vi "SV TDMS Read Spectrum Info.vi"(0 "tdms file":refnum<k34>, 5 "group name in":string, 7 "channel name in":string, 11 "error in":errorcluster) -> (4 "tdms file out":refnum<k34>, 6 "group name out":string, 8 "channel name out":string, 14 "spectrum info":T1 {"x-axis units" items=["Time (s)"=0, "Frequency-CB (Hz)"=1, "Frequency-CPB (Hz)"=1248, "Frequency-Arbitrary (Hz)"=2357, "Quefrency (s)"=2, "Revolutions (rev)"=3, "Order"=4, "Speed (RPM)"=11, "Speed (rad/s)"=21, "Index"=65535]; "weighting filter" items=["Linear", "A-weighting", "B-weighting", "C-weighting", "ITU-R 468-4", "Dolby", "CCITT", "C-message", "Wb", "Wc", "Wd", "We", "Wf", "Wh", "Wj", "Wk", "Wm", "AES17 20 kHz lowpass", "AES17 40 kHz lowpass", "AES17 20 kHz highpass", "AES17 40 kHz highpass"]; "dB reference [EU]" format="%.2f"; "engineering units" items=["custom..."=0, "V"=1, "A"=21, "C"=30, "pC"=31, "s"=32, "-"=29, "Pa"=2, "N"=20, "g"=3, "m/s^2"=4, "m/s"=5, "m"=6, "mm/s"=12, "mm"=13, "micron/s"=14, "micron"=15, "in/s^2"=7, "in/s"=8, "in"=9, "mil/s"=10, "mil"=11, "rad/s^2"=16, "rad/s"=17, "rad"=18, "deg/s^2"=26, "deg/s"=27, "deg"=28, "RPM"=22, "cycle/s^2"=23, "Hz"=24, "cycle"=25, "strain"=19]; "spectral info"."window" items=["None "=0, "Hanning"=1, "Hamming"=2, "Blackman-Harris"=3, "Exact Blackman"=4, "Blackman"=5, "Flat Top"=6, "4 Term B-Harris "=7, "7 Term B-Harris"=8, "Low Sidelobe"=9, "Force - Exponential"=10, "Gaussian"=62]}, 15 "error out":errorcluster)   [LabVIEW 2017]
uses:
  <vilib>/addons/_NISVFA/_Shared subVIs/Controls/svc_Spectrum Info.ctl
  <vilib>/addons/_NISVFA/_Shared subVIs/Controls/svc_X-Axis Units.ctl
  <vilib>/addons/_NISVFA/_Shared subVIs/Controls/svc_Spectrum Type.ctl
  <vilib>/addons/_NISVFA/_Shared subVIs/Controls/svc_Engineering Units Text Ring.ctl
  <vilib>/addons/_NISVFA/_Shared subVIs/Controls/svc_Weighting Filter Text Ring.ctl
  <vilib>/addons/_NISVFA/_Shared subVIs/Controls/svc_Complimentary Spectrum Units.ctl
  <vilib>/addons/_NISVFA/_Shared subVIs/Controls/NI Channel Properties.ctl
  <vilib>/addons/_NISVFA/_Shared subVIs/Controls/SV Channel Properties.ctl
  <vilib>/addons/_NISVFA/_Shared subVIs/Common/svc_Get Weighting Enum and Labels.vi
  <vilib>/addons/_NISVFA/_Shared subVIs/Common/svc_Unit Label Lexical Class.vi
  <vilib>/addons/_NISVFA/_Shared subVIs/Common/svc_Format Value (DBL).vi
  <vilib>/addons/_NISVFA/_Shared subVIs/Spectrum Info/sfva_Get SV Info from Spectrum Info Description.vi
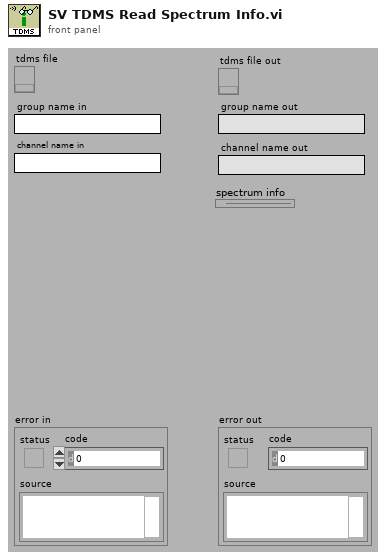
[diagram p1: front panel]
types:
  T1 = typedef "svc_Spectrum Info.ctl" = cluster{"channel name":string, "description":string, "x-axis units":T2, "spectral info":cluster{"spectrum type":T3, "linear/dB":enum16{"linear", "dB"}, "window":u16, "window size":i32, "FFT size":i32}, "engineering units":T4, "custom label":string, "dB reference [EU]":dbl, "peak units":enum16{"rms", "peak", "peak-peak"}, "weighting filter":T5, "spectral density?":bool, "unit label":string, "spectrum skewed?":bool, "complimentary spectrum units":T6}
  T2 = typedef "svc_X-Axis Units.ctl" = u16
  T3 = typedef "svc_Spectrum Type.ctl" = enum16{"FFT Spectrum [complex]", "Amplitude [Magnitude]", "Power [Magnitude^2]", "Cross Spectrum [complex]", "Frequency Response [Complex]"}
  T4 = typedef "svc_Engineering Units Text Ring.ctl" = u16
  T5 = typedef "svc_Weighting Filter Text Ring.ctl" = u16
  T6 = typedef "svc_Complimentary Spectrum Units.ctl" = enum16{"none", "radians", "degrees", "cycles", "imaginary"}
  T7 = typedef "NI Channel Properties.ctl" = u16
  T8 = typedef "NI Function Info.ctl" = cluster{"function type":T9, "function subtype":T10, "X-dimension":T2}
  T9 = typedef "NI Function Type.ctl" = u16
  T10 = typedef "NI Function SubType.ctl" = u16
  T11 = enum16{"No averaging", "Vector averaging", "RMS averaging", "Peak hold"}
  T12 = typedef "SV Channel Properties.ctl" = u16
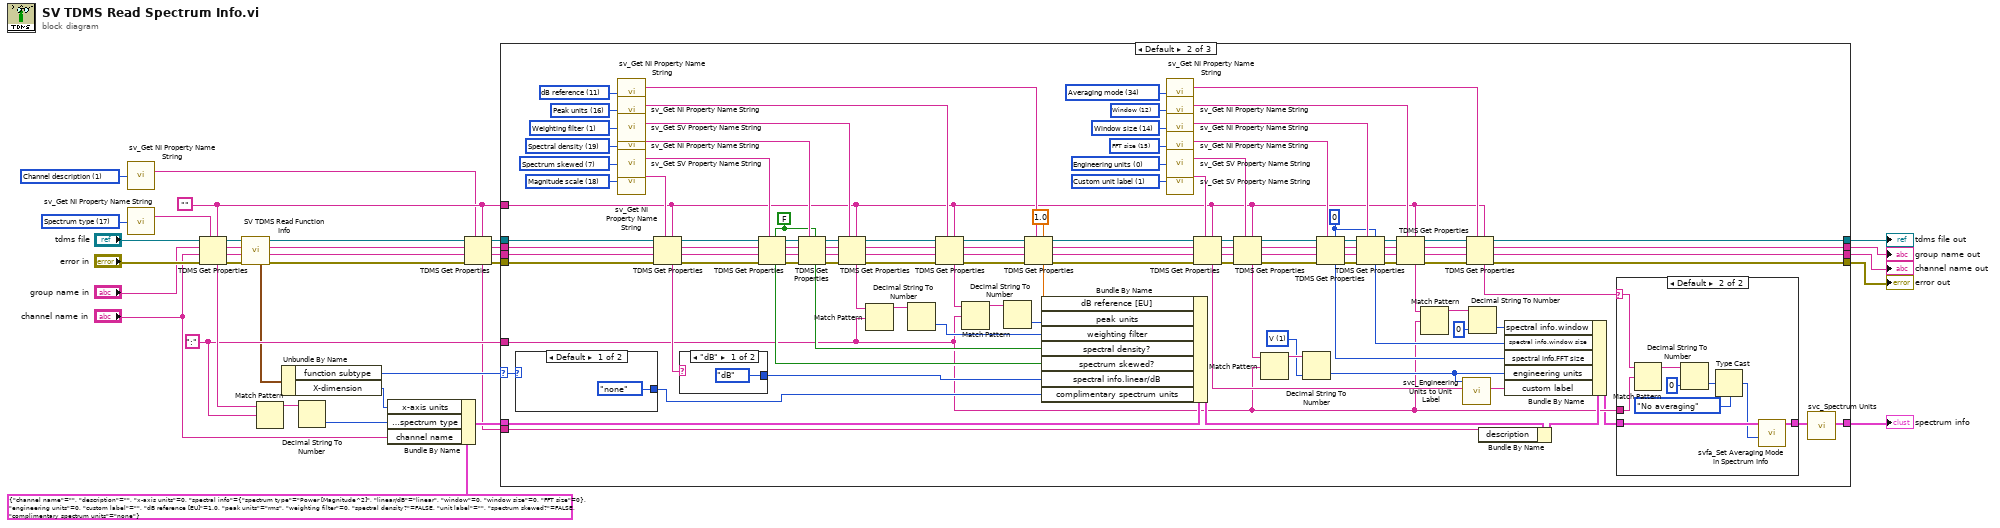
[diagram p0: block diagram]
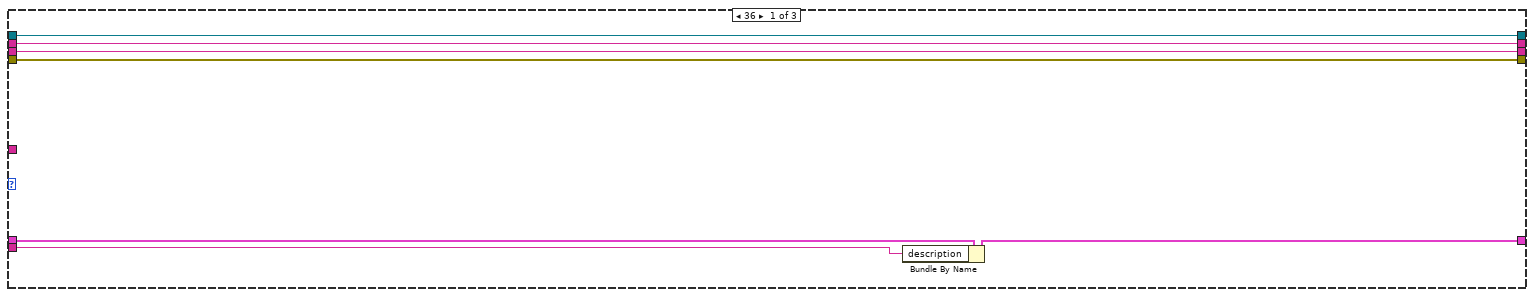
[diagram p2: hidden frame]
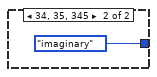
[diagram p4: hidden frame]
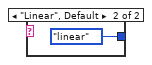
[diagram p5: hidden frame]
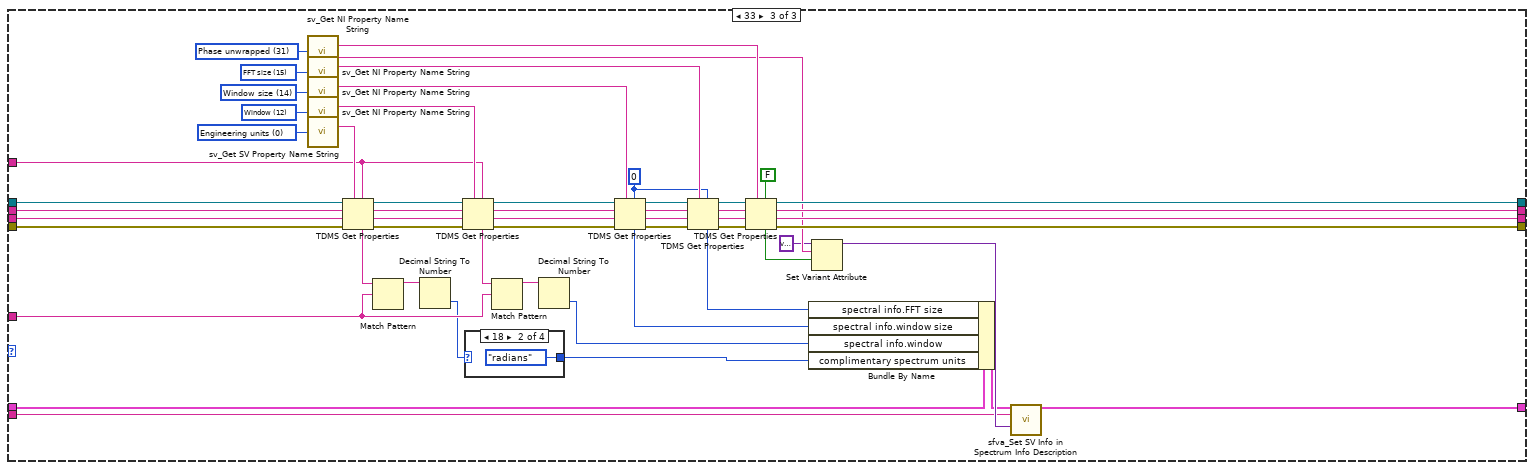
[diagram p6: hidden frame]
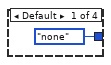
[diagram p7: hidden frame]
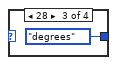
[diagram p8: hidden frame]
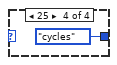
[diagram p9: hidden frame]
diagram:
  w6 = T7 1 items=["Channel name", "Channel description", "Axis label", "Unit string", "Waveform X-axis label", "Waveform X-axis unit string", "x0", "dx", "Number of samples", "X channel", "Filter settled", "dB reference", "Window", "Window parameter", "Window size", "FFT size", "Peak units", "Spectrum type", "Magnitude scale", "Spectral density", "Sensor sensitivity (mV/EU)", "X-axis dimension", "LabVIEW datatype", "Function type", "Function subtype", "X values", "Independent channel", "Column index", "Collection name", "Collection ID", "X Columns", "Phase unwrapped"] ("property")
  w18 = ":" ("regular expression")
  w7 = "" ("TDMS property name")
  w32 = T7 17 items=["Channel name", "Channel description", "Y-axis label", "Y-axis unit string", "X-axis label", "X-axis unit string", "x0", "dx", "Number of samples", "X channel", "Filter settled", "dB reference", "Window", "Window parameter", "Window size", "FFT size", "Peak units", "Spectrum type", "Magnitude scale", "Spectral density"] ("property")
  n1 = call <vilib>:"sv_Get NI Property Name String.vi"("property"=w6) -> ("TDMS property name"=w5:string)  [unwired: 13 in, 1 out]
  n2 = call <vilib>:"sv_Get NI Property Name String.vi"("property"=w32) -> ("TDMS property name"=w31:string)  [unwired: 13 in, 1 out]
  n3 = TDMS Get Properties(5:w7, 7:w31, 8:"error in", 9:"channel name in", 10:"group name in", 11:"tdms file") -> (0:w21:errorcluster, 1:w20:string, 2:w19:string, 3:w22:refnum<k34>, 4:w30:string)  [unwired: 1 out]
  n4 = call <vilib>:"SV TDMS Read Function Info.vi"("error in (no error)"=w21, "channel name"=w20, "group name"=w19, "tdms file in"=w22) -> ("error out"=w14:errorcluster, "channel name out"=w13:string, "group name out"=w12:string, "tdms file out"=w11:refnum<k34>, "function info"=w17:T8)  [unwired: 2 in, 1 out]
  n5 = Match Pattern(string=w30, regular expression=w18) -> (before substring=w29:string)  [unwired: 1 in, 3 out]
  n6 = Unbundle By Name(w17) -> ("function subtype"=w16:T10, "X-dimension"=w15:T2)
  n7 = Decimal String To Number(string=w29) -> (number=w28:i32)  [unwired: 2 in, 1 out]
  n8 = Bundle By Name(cluster=T1 {"channel name"="", "description"="", "x-axis units"=0, "spectral info"={"spectrum type"=enum."Power [Magnitude^2]", "linear/dB"=enum."linear", "window"=0, "window size"=0, "FFT size"=0}, "engineering units"=0, "custom label"="", "dB reference [EU]"=1.0, "peak units"=enum."rms", "weighting filter"=0, "spectral density?"=FALSE, "unit label"="", "spectrum skewed?"=FALSE, "complimentary spectrum units"=enum."none"} ("spectrum info in"), "x-axis units"=w15, "spectral info.spectrum type"=w28, "channel name"="channel name in") -> (w27:T1)
  n9 = TDMS Get Properties(5:w7, 7:w5, 8:w14, 9:w13, 10:w12, 11:w11) -> (0:w1:errorcluster, 1:w8:string, 2:w9:string, 3:w10:refnum<k34>, 4:w2:string)  [unwired: 1 out]
  n10 = case shown="Default" w16 {
    selector: w16 -> [_ w62 _]
    tunnel: [w43 w52 w185] -> w36
    tunnel: [w42 w53 w184] -> w35
    tunnel: [w41 w54 w183] -> w34
    tunnel: [w40 w55 w182] -> w33
    tunnel: w10 -> [w43 w126 w226]
    tunnel: w9 -> [w42 w127 w225]
    tunnel: w8 -> [w41 w128 w224]
    tunnel: w1 -> [w40 w129 w223]
    tunnel: w7 -> [_ w50 w201]
    tunnel: w18 -> [_ w48 w198]
    tunnel: w27 -> [w39 w77 w195]
    tunnel: [w38 w69 w174] -> w3
    tunnel: w2 -> [w37 w63 w173]
    frame 36 {
      n11 = Bundle By Name(cluster=w39, "description"=w37) -> (w38:T1)
    }
    frame Default {
      w44 = T4 1 items=["custom..."=0, "V"=1, "A"=21, "C"=30, "pC"=31, "s"=32, "-"=29, "Pa"=2, "N"=20, "g"=3, "m/s^2"=4, "m/s"=5, "m"=6, "mm/s"=12, "mm"=13, "micron/s"=14, "micron"=15, "in/s^2"=7, "in/s"=8, "in"=9, "mil/s"=10, "mil"=11, "rad/s^2"=16, "rad/s"=17, "rad"=18, "deg/s^2"=26, "deg/s"=27, "deg"=28, "RPM"=22, "cycle/s^2"=23, "Hz"=24, "cycle"=25, "strain"=19] ("engineering units")
      w60 = T7 34 items=["Channel name", "Channel description", "Axis label", "Unit string", "Waveform X-axis label", "Waveform X-axis unit string", "x0", "dx", "Number of samples", "X channel", "Filter settled", "dB reference", "Window", "Window parameter", "Window size", "FFT size", "Peak units", "Spectrum type", "Magnitude scale", "Spectral density", "Sensor sensitivity (mV/EU)", "X-axis dimension", "LabVIEW datatype", "Function type", "Function subtype", "X values", "Independent channel", "Column index", "Collection name", "Collection ID", "X Columns", "Phase unwrapped", "Sensor type", "Sensor maximum", "Averaging mode"] ("property")
      w97 = T7 18 items=["Channel name", "Channel description", "Y-axis label", "Y-axis unit string", "X-axis label", "X-axis unit string", "x0", "dx", "Number of samples", "X channel", "Filter settled", "dB reference", "Window", "Window parameter", "Window size", "FFT size", "Peak units", "Spectrum type", "Magnitude scale", "Spectral density"] ("property")
      w98 = T12 0 items=["Engineering units", "Weighting filter", "Pregain", "Octave standard", "Octave bandwidth", "Octave low band", "Octave high band", "Spectrum skewed"] ("property")
      w103 = T7 15 items=["Channel name", "Channel description", "Y-axis label", "Y-axis unit string", "X-axis label", "X-axis unit string", "x0", "dx", "Number of samples", "X channel", "Filter settled", "dB reference", "Window", "Window parameter", "Window size", "FFT size", "Peak units", "Spectrum type", "Magnitude scale", "Spectral density"] ("property")
      w104 = T7 14 items=["Channel name", "Channel description", "Y-axis label", "Y-axis unit string", "X-axis label", "X-axis unit string", "x0", "dx", "Number of samples", "X channel", "Filter settled", "dB reference", "Window", "Window parameter", "Window size", "FFT size", "Peak units", "Spectrum type", "Magnitude scale", "Spectral density"] ("property")
      w105 = T7 12 items=["Channel name", "Channel description", "Y-axis label", "Y-axis unit string", "X-axis label", "X-axis unit string", "x0", "dx", "Number of samples", "X channel", "Filter settled", "dB reference", "Window", "Window parameter", "Window size", "FFT size", "Peak units", "Spectrum type", "Magnitude scale", "Spectral density"] ("property")
      w109 = T12 1 items=["Engineering units", "Custom unit label", "Weighting filter", "Pregain", "Octave standard", "Octave bandwidth", "Octave low band", "Octave high band", "Spectrum skewed"] ("property")
      w110 = T7 11 items=["Channel name", "Channel description", "Y-axis label", "Y-axis unit string", "X-axis label", "X-axis unit string", "x0", "dx", "Number of samples", "X channel", "Filter settled", "dB reference", "Window", "Window parameter", "Window size", "FFT size", "Peak units", "Spectrum type", "Magnitude scale", "Spectral density"] ("property")
      w111 = T7 16 items=["Channel name", "Channel description", "Y-axis label", "Y-axis unit string", "X-axis label", "X-axis unit string", "x0", "dx", "Number of samples", "X channel", "Filter settled", "dB reference", "Window", "Window parameter", "Window size", "FFT size", "Peak units", "Spectrum type", "Magnitude scale", "Spectral density"] ("property")
      w113 = T7 19 items=["Channel name", "Channel description", "Y-axis label", "Y-axis unit string", "X-axis label", "X-axis unit string", "x0", "dx", "Number of samples", "X channel", "Filter settled", "dB reference", "Window", "Window parameter", "Window size", "FFT size", "Peak units", "Spectrum type", "Magnitude scale", "Spectral density"] ("property")
      w115 = T12 7 items=["Engineering units", "Weighting filter", "Pregain", "Octave standard", "Octave bandwidth", "Octave low band", "Octave high band", "Spectrum skewed"] ("property")
      w116 = T12 1 items=["Engineering units", "Weighting filter", "Pregain", "Octave standard", "Octave bandwidth", "Octave low band", "Octave high band", "Spectrum skewed"] ("property")
      w89 = 0 ("FFT size")
      w95 = FALSE ("spectrum skewed?")
      n12 = case shown="Default" w62 {
        tunnel: [svc_Complimentary_Spectrum_Units."none" ("complimentary spectrum units") svc_Complimentary_Spectrum_Units."imaginary" ("complimentary spectrum units")] -> w61
        frame Default {
        }
        frame 34, 35, 345 {
        }
      }
      n13 = call <vilib>:"sv_Get NI Property Name String.vi"("property"=w110) -> ("TDMS property name"=w107:string)  [unwired: 13 in, 1 out]
      n14 = call <vilib>:"sv_Get NI Property Name String.vi"("property"=w111) -> ("TDMS property name"=w106:string)  [unwired: 13 in, 1 out]
      n15 = call <vilib>:"sv_Get SV Property Name String.vi"("property"=w116) -> ("TDMS property name"=w117:string)  [unwired: 13 in, 1 out]
      n16 = call <vilib>:"sv_Get NI Property Name String.vi"("property"=w113) -> ("TDMS property name"=w112:string)  [unwired: 13 in, 1 out]
      n17 = call <vilib>:"sv_Get SV Property Name String.vi"("property"=w115) -> ("TDMS property name"=w114:string)  [unwired: 13 in, 1 out]
      n18 = call <vilib>:"sv_Get NI Property Name String.vi"("property"=w97) -> ("TDMS property name"=w96:string)  [unwired: 13 in, 1 out]
      n19 = TDMS Get Properties(5:w50, 7:w96, 8:w129, 9:w128, 10:w127, 11:w126) -> (0:w122:errorcluster, 1:w123:string, 2:w124:string, 3:w125:refnum<k34>, 4:w88:string)  [unwired: 1 out]
      n20 = case shown="\"dB\"" w88 {
        tunnel: [enum16{"linear", "dB"}."dB" ("spectral info.linear/dB") enum16{"linear", "dB"}."linear" ("spectral info.linear/dB")] -> w87
        frame "dB" {
        }
        frame "Linear", Default {
        }
      }
      n21 = TDMS Get Properties(5:w95, 7:w114, 8:w122, 9:w123, 10:w124, 11:w125) -> (0:w118:errorcluster, 1:w119:string, 2:w120:string, 3:w121:refnum<k34>, 4:w86:bool)  [unwired: 1 out]
      n22 = TDMS Get Properties(5:w95, 7:w112, 8:w118, 9:w119, 10:w120, 11:w121) -> (0:w142:errorcluster, 1:w141:string, 2:w140:string, 3:w139:refnum<k34>, 4:w85:bool)  [unwired: 1 out]
      n23 = TDMS Get Properties(5:w50, 7:w117, 8:w142, 9:w141, 10:w140, 11:w139) -> (0:w143:errorcluster, 1:w144:string, 2:w145:string, 3:w146:refnum<k34>, 4:w83:string)  [unwired: 1 out]
      n24 = Match Pattern(string=w83, regular expression=w48) -> (before substring=w84:string)  [unwired: 1 in, 3 out]
      n25 = Decimal String To Number(string=w84) -> (number=w79:i32)  [unwired: 2 in, 1 out]
      n26 = TDMS Get Properties(5:w50, 7:w106, 8:w143, 9:w144, 10:w145, 11:w146) -> (0:w138:errorcluster, 1:w137:string, 2:w136:string, 3:w135:refnum<k34>, 4:w81:string)  [unwired: 1 out]
      n27 = Match Pattern(string=w81, regular expression=w48) -> (before substring=w82:string)  [unwired: 1 in, 3 out]
      n28 = Decimal String To Number(string=w82) -> (number=w80:i32)  [unwired: 2 in, 1 out]
      n29 = TDMS Get Properties(5:1.0 ("x"), 7:w107, 8:w138, 9:w137, 10:w136, 11:w135) -> (0:w131:errorcluster, 1:w132:string, 2:w133:string, 3:w134:refnum<k34>, 4:w78:dbl)  [unwired: 1 out]
      n30 = Bundle By Name(cluster=w77, "dB reference [EU]"=w78, "peak units"=w80, "weighting filter"=w79, "spectral density?"=w85, "spectrum skewed?"=w86, "spectral info.linear/dB"=w87, "complimentary spectrum units"=w61) -> (w65:T1)
      n31 = call <vilib>:"sv_Get NI Property Name String.vi"("property"=w60) -> ("TDMS property name"=w51:string)  [unwired: 13 in, 1 out]
      n32 = call <vilib>:"sv_Get NI Property Name String.vi"("property"=w105) -> ("TDMS property name"=w100:string)  [unwired: 13 in, 1 out]
      n33 = call <vilib>:"sv_Get NI Property Name String.vi"("property"=w104) -> ("TDMS property name"=w101:string)  [unwired: 13 in, 1 out]
      n34 = call <vilib>:"sv_Get NI Property Name String.vi"("property"=w103) -> ("TDMS property name"=w102:string)  [unwired: 13 in, 1 out]
      n35 = call <vilib>:"sv_Get SV Property Name String.vi"("property"=w98) -> ("TDMS property name"=w99:string)  [unwired: 13 in, 1 out]
      n36 = call <vilib>:"sv_Get SV Property Name String.vi"("property"=w109) -> ("TDMS property name"=w108:string)  [unwired: 13 in, 1 out]
      n37 = TDMS Get Properties(5:w50, 7:w108, 8:w131, 9:w132, 10:w133, 11:w134) -> (0:w147:errorcluster, 1:w130:string, 2:w148:string, 3:w149:refnum<k34>, 4:w67:string)  [unwired: 1 out]
      n38 = TDMS Get Properties(5:w50, 7:w99, 8:w147, 9:w130, 10:w148, 11:w149) -> (0:w150:errorcluster, 1:w151:string, 2:w152:string, 3:w153:refnum<k34>, 4:w75:string)  [unwired: 1 out]
      n39 = Match Pattern(string=w75, regular expression=w48) -> (before substring=w76:string)  [unwired: 1 in, 3 out]
      n40 = Decimal String To Number(string=w76, default (0L)=w44) -> (number=w68:u16)  [unwired: 1 in, 1 out]
      n41 = TDMS Get Properties(5:w89, 7:w102, 8:w150, 9:w151, 10:w152, 11:w153) -> (0:w154:errorcluster, 1:w155:string, 2:w156:string, 3:w157:refnum<k34>, 4:w74:i32)  [unwired: 1 out]
      n42 = TDMS Get Properties(5:w89, 7:w101, 8:w154, 9:w155, 10:w156, 11:w157) -> (0:w90:errorcluster, 1:w91:string, 2:w92:string, 3:w93:refnum<k34>, 4:w73:i32)  [unwired: 1 out]
      n43 = TDMS Get Properties(5:w50, 7:w100, 8:w90, 9:w91, 10:w92, 11:w93) -> (0:w56:errorcluster, 1:w57:string, 2:w58:string, 3:w59:refnum<k34>, 4:w71:string)  [unwired: 1 out]
      n44 = Match Pattern(string=w71, regular expression=w48) -> (before substring=w72:string)  [unwired: 1 in, 3 out]
      n45 = call <vilib>:"svc_Engineering Units to Unit Label.vi"("custom label"=w67, "engineering units"=w68) -> ("unit label"=w66:string)  [unwired: 8 in, 1 out]
      n46 = TDMS Get Properties(5:w50, 7:w51, 8:w56, 9:w57, 10:w58, 11:w59) -> (0:w55:errorcluster, 1:w54:string, 2:w53:string, 3:w52:refnum<k34>, 4:w49:string)  [unwired: 1 out]
      n47 = Decimal String To Number(string=w72, default (0L)=u16 0 ("spectral info.window")) -> (number=w70:u16)  [unwired: 1 in, 1 out]
      n48 = Bundle By Name(cluster=w65, "description"=w63) -> (w64:T1)
      n49 = Bundle By Name(cluster=w64, "spectral info.window"=w70, "spectral info.window size"=w73, "spectral info.FFT size"=w74, "engineering units"=w68, "custom label"=w66) -> (w47:T1)
      n50 = case shown="Default" w49 {
        selector: w49 -> [_ w166]
        tunnel: w48 -> [_ w165]
        tunnel: w47 -> [w158 w161]
        tunnel: [w158 w159] -> w46
        frame "" {
        }
        frame Default {
          n51 = Match Pattern(string=w166, regular expression=w165) -> (before substring=w167:string)  [unwired: 1 in, 3 out]
          n52 = Decimal String To Number(string=w167, default (0L)=u16 0 ("default (0 I32)")) -> (number=w163:u16)  [unwired: 1 in, 1 out]
          n53 = Type Cast(type=T11."No averaging" ("averaging mode 2"), x=w163) -> (*(type *) &x=w160:T11)
          n54 = call <vilib>:"svfa_Set Averaging Mode in Spectrum Info.vi"("averaging mode"=w160, "spectrum info in"=w161) -> ("spectrum info out"=w159:T1)  [unwired: 8 in, 1 out]
        }
      }
      n55 = call <vilib>:"svc_Spectrum Units.vi"("spectrum info in"=w46) -> ("spectrum info out"=w69:T1)  [unwired: 3 in, 3 out]
    }
    frame 33 {
      w181 = T7 31 items=["Channel name", "Channel description", "Axis label", "Unit string", "Waveform X-axis label", "Waveform X-axis unit string", "x0", "dx", "Number of samples", "X channel", "Filter settled", "dB reference", "Window", "Window parameter", "Window size", "FFT size", "Peak units", "Spectrum type", "Magnitude scale", "Spectral density", "Sensor sensitivity (mV/EU)", "X-axis dimension", "LabVIEW datatype", "Function type", "Function subtype", "X values", "Independent channel", "Column index", "Collection name", "Collection ID", "X Columns", "Phase unwrapped"] ("property")
      w204 = T7 15 items=["Channel name", "Channel description", "Y-axis label", "Y-axis unit string", "X-axis label", "X-axis unit string", "x0", "dx", "Number of samples", "X channel", "Filter settled", "dB reference", "Window", "Window parameter", "Window size", "FFT size", "Peak units", "Spectrum type", "Magnitude scale", "Spectral density"] ("property")
      w205 = T7 14 items=["Channel name", "Channel description", "Y-axis label", "Y-axis unit string", "X-axis label", "X-axis unit string", "x0", "dx", "Number of samples", "X channel", "Filter settled", "dB reference", "Window", "Window parameter", "Window size", "FFT size", "Peak units", "Spectrum type", "Magnitude scale", "Spectral density"] ("property")
      w208 = T7 12 items=["Channel name", "Channel description", "Y-axis label", "Y-axis unit string", "X-axis label", "X-axis unit string", "x0", "dx", "Number of samples", "X channel", "Filter settled", "dB reference", "Window", "Window parameter", "Window size", "FFT size", "Peak units", "Spectrum type", "Magnitude scale", "Spectral density"] ("property")
      w209 = T12 0 items=["Engineering units", "Custom unit label", "Weighting filter", "Pregain", "Octave standard", "Octave bandwidth", "Octave low band", "Octave high band", "Spectrum skewed"] ("SV property")
      w202 = 0 ("FFT size")
      n56 = call <vilib>:"sv_Get NI Property Name String.vi"("property"=w181) -> ("TDMS property name"=w180:string, "WDT attribute name"=w178:string)  [unwired: 13 in]
      n57 = call <vilib>:"sv_Get NI Property Name String.vi"("property"=w204) -> ("TDMS property name"=w203:string)  [unwired: 13 in, 1 out]
      n58 = call <vilib>:"sv_Get NI Property Name String.vi"("property"=w205) -> ("TDMS property name"=w206:string)  [unwired: 13 in, 1 out]
      n59 = call <vilib>:"sv_Get NI Property Name String.vi"("property"=w208) -> ("TDMS property name"=w207:string)  [unwired: 13 in, 1 out]
      n60 = call <vilib>:"sv_Get SV Property Name String.vi"("property"=w209) -> ("TDMS property name"=w210:string)  [unwired: 13 in, 1 out]
      n61 = TDMS Get Properties(5:w201, 7:w210, 8:w223, 9:w224, 10:w225, 11:w226) -> (0:w211:errorcluster, 1:w212:string, 2:w214:string, 3:w213:refnum<k34>, 4:w200:string)  [unwired: 1 out]
      n62 = Match Pattern(string=w200, regular expression=w198) -> (before substring=w196:string)  [unwired: 1 in, 3 out]
      n63 = Decimal String To Number(string=w196) -> (number=w191:i32)  [unwired: 2 in, 1 out]
      n64 = TDMS Get Properties(5:w201, 7:w207, 8:w211, 9:w212, 10:w214, 11:w213) -> (0:w215:errorcluster, 1:w216:string, 2:w217:string, 3:w218:refnum<k34>, 4:w199:string)  [unwired: 1 out]
      n65 = case shown="18" w191 {
        tunnel: [svc_Complimentary_Spectrum_Units."none" ("complimentary spectrum units") svc_Complimentary_Spectrum_Units."radians" ("complimentary spectrum units") svc_Complimentary_Spectrum_Units."degrees" ("complimentary spectrum units") svc_Complimentary_Spectrum_Units."cycles" ("complimentary spectrum units")] -> w190
        frame Default {
        }
        frame 18 {
        }
        frame 28 {
        }
        frame 25 {
        }
      }
      n66 = Match Pattern(string=w199, regular expression=w198) -> (before substring=w197:string)  [unwired: 1 in, 3 out]
      n67 = Decimal String To Number(string=w197) -> (number=w194:i32)  [unwired: 2 in, 1 out]
      n68 = TDMS Get Properties(5:w202, 7:w206, 8:w215, 9:w216, 10:w217, 11:w218) -> (0:w219:errorcluster, 1:w220:string, 2:w221:string, 3:w222:refnum<k34>, 4:w193:i32)  [unwired: 1 out]
      n69 = TDMS Get Properties(5:w202, 7:w203, 8:w219, 9:w220, 10:w221, 11:w222) -> (0:w189:errorcluster, 1:w188:string, 2:w187:string, 3:w186:refnum<k34>, 4:w192:i32)  [unwired: 1 out]
      n70 = TDMS Get Properties(5:FALSE ("spectrum skewed?"), 7:w180, 8:w189, 9:w188, 10:w187, 11:w186) -> (0:w182:errorcluster, 1:w183:string, 2:w184:string, 3:w185:refnum<k34>, 4:w177:bool)  [unwired: 1 out]
      n71 = Bundle By Name(cluster=w195, "spectral info.FFT size"=w192, "spectral info.window size"=w193, "spectral info.window"=w194, "complimentary spectrum units"=w190) -> (w175:T1)
      n72 = Set Variant Attribute(Variant=variant ("variant"), name=w178, value=w177) -> (Variant out=w176:variant)  [unwired: 1 in, 2 out]
      n73 = call <vilib>:"sfva_Set SV Info in Spectrum Info Description.vi"("spectrum info"=w175, "description"=w173, "SV Info"=w176) -> ("spectrum info"=w174:T1)  [unwired: 11 in, 1 out]
    }
  }
  "tdms file out" <- w36
  "group name out" <- w35
  "channel name out" <- w34
  "error out" <- w33
  "spectrum info" <- w3
